vi "MongoDB.Database.Drop.vi"(8 "error in (no error)":errorcluster, 11 "MongoDB.Database in":refnum<class "MongoDB.Database.lvclass">) -> (0 "error out":errorcluster, 3 "MongoDB.Database out":refnum<class "MongoDB.Database.lvclass">)   [LabVIEW 2014, in "MongoDB.Database.lvclass"]
uses:
  MongoDB.Database.lvclass
  MongoDB.Database.lvclass/MongoDB.Database.ctl
  C:/Users/Richard/Documents/GitHub/mongo-labview-driver/CSharp/bin/MongoDB.Driver.Legacy.dll
  CSharp/bin/MongoDB.Driver.Legacy.dll
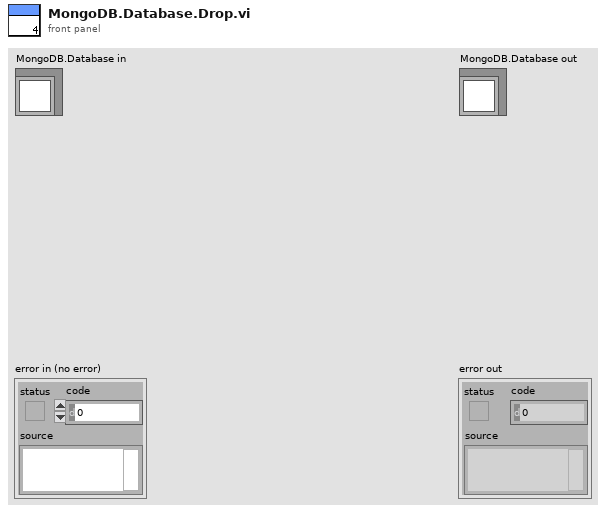
[diagram p1: front panel]
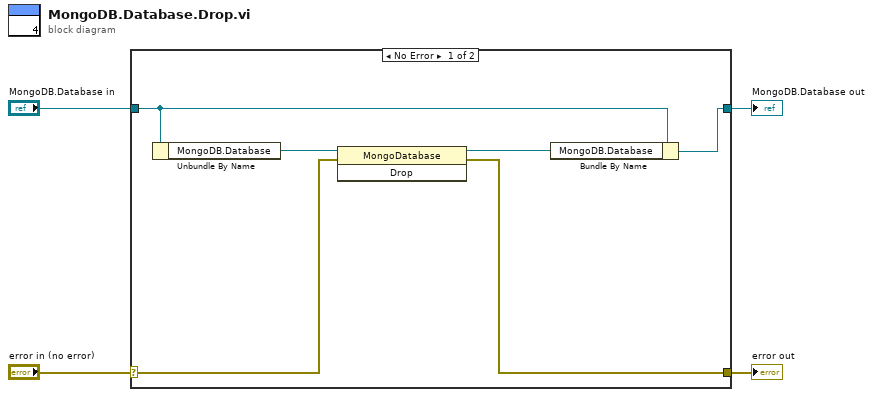
[diagram p0: block diagram]
diagram:
  n1 = case shown="No Error" "error in (no error)" {
    selector: "error in (no error)" -> [w9 w12]
    tunnel: [w8 w12] -> w3
    tunnel: [w5 w11] -> w1
    tunnel: "MongoDB.Database in" -> [w7 w11]
    frame No Error {
      n2 = Unbundle By Name(w7) -> ("MongoDB.Database"=w10:refnum<k24>)
      n3 = invoke class="MongoDatabase" method="Drop"(reference=w10, error in=w9) -> (reference out=w6:refnum<k24>, error out=w8:errorcluster)  [unwired: 1 in, 1 out]
      n4 = Bundle By Name(cluster=w7, "MongoDB.Database"=w6) -> (w5:refnum<class "MongoDB.Database.lvclass">)
    }
    frame Error {
    }
  }
  "error out" <- w3
  "MongoDB.Database out" <- w1
